vi "Calc - RhoFuel.vi"(11 "TFFT":dbl) -> (3 "RhoFuel":dbl)   [LabVIEW 2018, in "Controller (Host).lvlib"]
uses:
  Controller (Host).lvlib
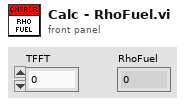
[diagram p1: front panel]
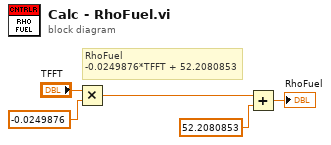
[diagram p0: block diagram]
diagram:
  # "RhoFuel\n-0.0249876*TFFT + 52.2080853"
  n1 = Multiply(x="TFFT", y=-0.0249876) -> (x*y=w3:dbl)
  n2 = Add(x=w3, y=52.2080853) -> (x+y=→"RhoFuel":dbl)
